vi "E-Time (mS).vi"(6 "Enter Start Time(mS)":u32 caption="Set Start Time (s)", 8 "error in (no error)":errorcluster, 9 "Reset":bool) -> (0 "error out":errorcluster, 1 "Elapsed Time (mS)":u32, 4 "Time Since Last Run(mS)":u32)   [LabVIEW 2016]
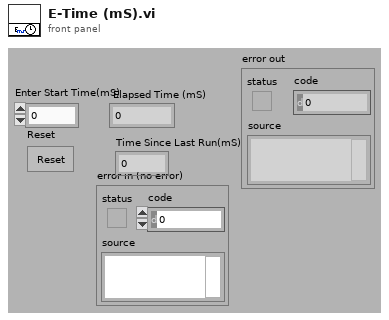
[diagram p1: front panel]
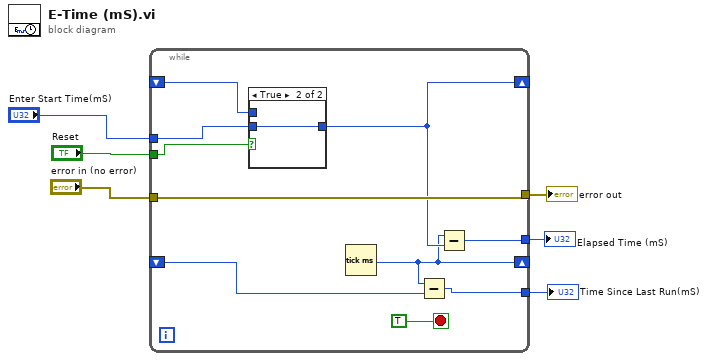
[diagram p0: block diagram]
diagram:
  n1 = while {
    tunnel: "Reset" -> [w10]
    tunnel: "error in (no error)" -> [w9]
    tunnel: [w9] -> w3
    tunnel: [w15] -> w2
    tunnel: "Enter Start Time(mS)" -> [w12]
    shift-right: [w8] -> _
    shift-left: _ -> [w11]
    tunnel: [w13] -> w6
    shift-right: [w7] -> _
    shift-left: _ -> [w16]
    stop <- TRUE stop-if-true
    n2 = case shown="True" w10 {
      tunnel: [w17 w18] -> w8
      tunnel: w12 -> [_ w18]
      tunnel: w11 -> [w17 _]
      frame False {
      }
      frame True {
      }
    }
    n3 = Tick Count (ms)() -> (millisecond timer value=w7:u32)
    n4 = Subtract(x=w7, y=w16) -> (x-y=w15:u32)
    n5 = Subtract(x=w7, y=w8) -> (x-y=w13:u32)
  }
  "Elapsed Time (mS)" <- w6
  "error out" <- w3
  "Time Since Last Run(mS)" <- w2
